vi "parse gentec acquire string.vi"(11 "Acquisition String":string) -> (0 "AcqOkCh2":bool, 1 "AcqOkCh1":bool, 2 "Channel 2 value":dbl, 3 "Channel 1 value":dbl)   [LabVIEW 2020, in "Gentec Slink.lvclass"]
uses:
  Gentec Slink.lvclass
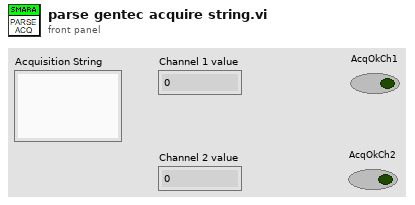
[diagram p1: front panel]
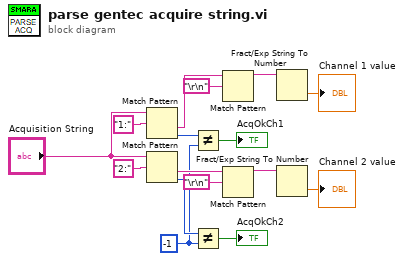
[diagram p0: block diagram]
diagram:
  w2 = -1
  n1 = Match Pattern(string="Acquisition String", regular expression="1:") -> (after substring=w10:string, offset past match=w5:i32)  [unwired: 1 in, 2 out]
  n2 = Match Pattern(string="Acquisition String", regular expression="2:") -> (after substring=w15:string, offset past match=w3:i32)  [unwired: 1 in, 2 out]
  n3 = Not Equal?(x=w5, y=w2) -> (x != y?=→"AcqOkCh1":bool)
  n4 = Not Equal?(x=w3, y=w2) -> (x != y?=→"AcqOkCh2":bool)
  n5 = Match Pattern(string=w10, regular expression="\r\n") -> (before substring=w11:string)  [unwired: 1 in, 3 out]
  n6 = Match Pattern(string=w15, regular expression="\r\n") -> (before substring=w16:string)  [unwired: 1 in, 3 out]
  n7 = Fract/Exp String To Number(string=w11) -> (number=→"Channel 1 value":dbl)  [unwired: 3 in, 1 out]
  n8 = Fract/Exp String To Number(string=w16) -> (number=→"Channel 2 value":dbl)  [unwired: 3 in, 1 out]
